vi "ScopeTrigger.vi"(4 "range":i32=5, 5 "voltsLevel":dbl, 6 "timeout":i32, 7 "trigcond":enum16{"Raising", "Falling", "Either"}(ring), 8 "error in (no error)":errorcluster caption="错误输入（无错误）", 9 "trigsrc":T1(ring), 10 "trigtype":enum16{"edge", "pulse", "trasition"}(ring), 11 "handle":u64) -> (0 "error out":errorcluster caption="错误输出", 2 "function return":i32, 3 "handle out":u64)   [LabVIEW 2018]
doc: "Set Scope Trigger Configration."
uses:
  InstrumentsPlayground.lvlib
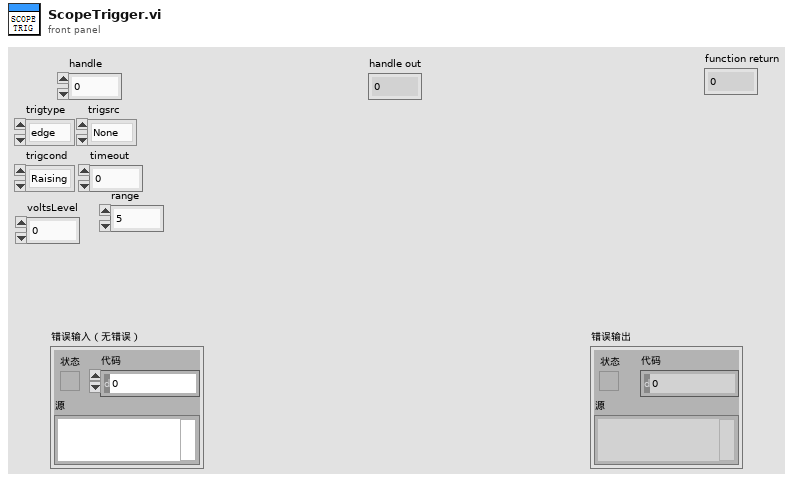
[diagram p1: front panel]
types:
  T1 = enum16{"None", "DetectorAnalogInCH1", "DetectorAnalogInCH2", "AnalogOut1", "AnalogOut2", "DetectorDigitalIn", "DigitalOut", "Manule", "External 1", "External 2", "DigitalIn"}
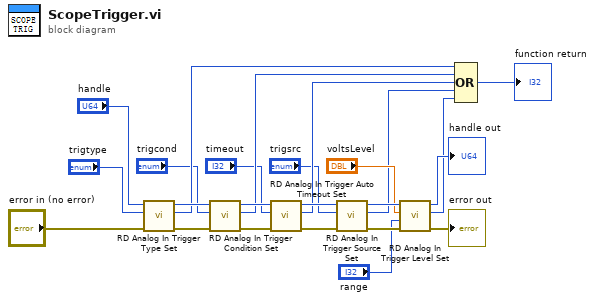
[diagram p0: block diagram]
diagram:
  n1 = call "RD Analog In Trigger Type Set.vi"("error in (no error)"="error in (no error)", "trigtype"="trigtype", "handle"="handle") -> ("error out"=w21:errorcluster, "function return"=w8:i32, "handle out"=w24:u64)  [unwired: 6 in]
  n2 = call "RD Analog In Trigger Condition Set.vi"("error in (no error)"=w21, "trigcond"="trigcond", "handle"=w24) -> ("error out"=w22:errorcluster, "function return"=w9:i32, "handle out"=w23:u64)  [unwired: 6 in]
  n3 = call "RD Analog In Trigger Auto Timeout Set.vi"("error in (no error)"=w22, "timeout"="timeout", "handle"=w23) -> ("error out"=w19:errorcluster, "function return"=w10:i32, "handle out"=w18:u64)  [unwired: 6 in]
  n4 = call "RD Analog In Trigger Source Set.vi"("error in (no error)"=w19, "trigsrc"="trigsrc", "handle"=w18) -> ("error out"=w16:errorcluster, "function return"=w11:i32, "handle out"=w17:u64)  [unwired: 6 in]
  n5 = call "RD Analog In Trigger Level Set.vi"("error in (no error)"=w16, "range"="range", "voltsLevel"="voltsLevel", "handle"=w17) -> ("error out"=→"error out":errorcluster, "function return"=w12:i32, "handle out"=→"handle out":u64)  [unwired: 5 in]
  n6 = Compound Arithmetic op=OR ("复合运算")(w8, w9, w10, w11, w12) -> (→"function return":i32)
